vi "Clear.vi"(8 "error in (no error)":errorcluster, 11 "VISA in":refnum<class "VISA.lvclass">) -> (0 "error out":errorcluster, 3 "VISA out":refnum<class "VISA.lvclass">)   [LabVIEW 2020, in "Low Level PSU With Tests.lvlib" / "VISA.lvclass"]
uses:
  VISA.lvclass
  VISA.lvclass/VISA.ctl
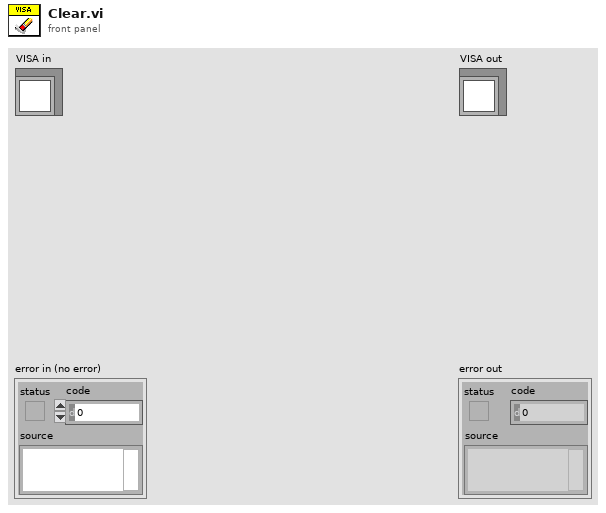
[diagram p1: front panel]
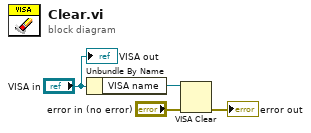
[diagram p0: block diagram]
diagram:
  n1 = Unbundle By Name("VISA in") -> ("VISA name"=w1:refnum<visa-resource-name>)
  n2 = VISA Clear(VISA resource name=w1, error in (no error)="error in (no error)") -> (error out=→"error out":errorcluster)  [unwired: 1 out]
  "VISA out" <- "VISA in"
